vi "ask_model_core.vi"(0 "agent_simple_qa in":refnum<class "agent_simple_qa.lvclass">, 5 "message":refnum<class "abstract_message_base.lvclass">, 11 "error in (no error)":errorcluster) -> (4 "agent_simple_qa out":refnum<class "agent_simple_qa.lvclass">, 6 "message_response":refnum<class "abstract_message_base.lvclass">, 15 "error out":errorcluster)   [LabVIEW 2020, in "agent_simple_qa.lvclass"]
uses:
  agent_simple_qa.lvclass
  models/abstract_message_base/abstract_message_base.lvclass
  agent_simple_qa.lvclass/agent_simple_qa.ctl
  models/abstract_llm_chatcompletion/abstract_llm_chatcompletion.lvclass
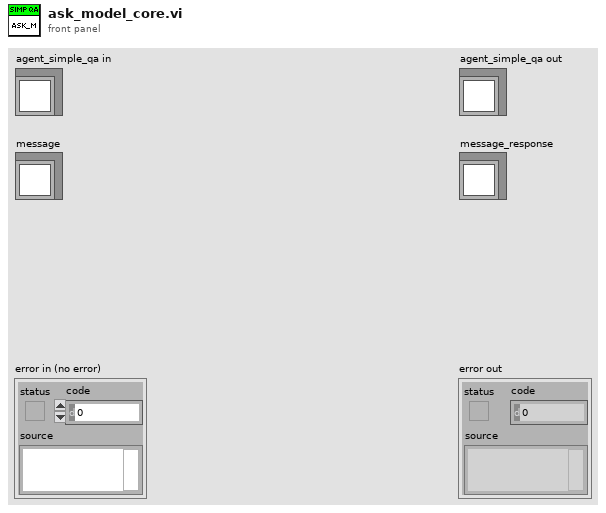
[diagram p1: front panel]
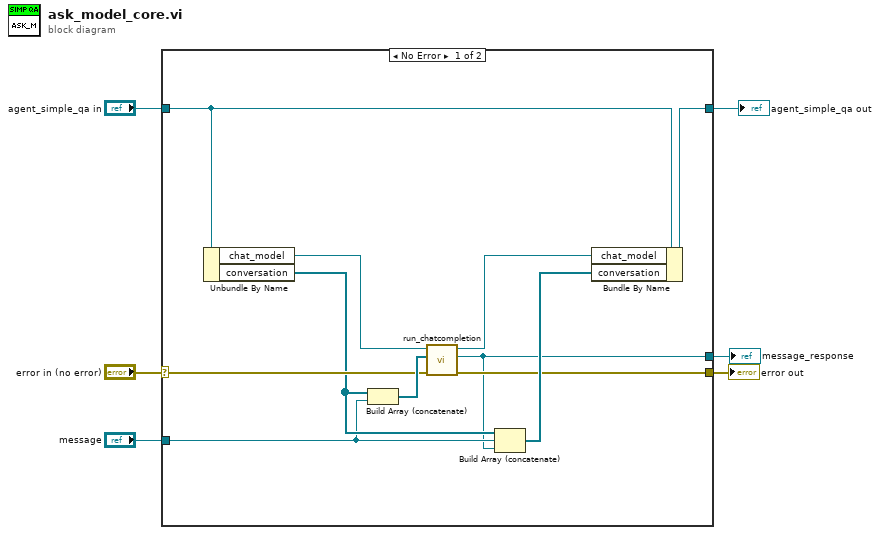
[diagram p0: block diagram]
diagram:
  n1 = case shown="No Error" "error in (no error)" {
    selector: "error in (no error)" -> [w13 w19]
    tunnel: [w8 w19] -> w5
    tunnel: [w16 w18] -> w3
    tunnel: "agent_simple_qa in" -> [w11 w18]
    tunnel: "message" -> [w9 _]
    tunnel: [w7 _] -> w2
    frame No Error {
      n2 = Unbundle By Name(w11) -> ("chat_model"=w12:refnum<class "abstract_llm_base.lvclass">, "conversation"=w10:refnum<class "abstract_message_base.lvclass">[])
      n3 = Build Array (concatenate)(w10, w9) -> (w15:refnum<class "abstract_message_base.lvclass">[])
      n4 = call "run_chatcompletion.vi"("error in (no error)"=w13, "Messages"=w15, "abstract_llm_chatcompletion in"=w12) -> ("error out"=w8:errorcluster, "Response"=w7:refnum<class "abstract_message_base.lvclass">, "abstract_llm_chatcompletion out"=w17:refnum<class "abstract_llm_base.lvclass">)  [unwired: 6 in]
      n5 = Build Array (concatenate)(w10, w9, w7) -> (w14:refnum<class "abstract_message_base.lvclass">[])
      n6 = Bundle By Name(cluster=w11, "chat_model"=w17, "conversation"=w14) -> (w16:refnum<class "agent_simple_qa.lvclass">)
    }
    frame Error {
    }
  }
  "error out" <- w5
  "agent_simple_qa out" <- w3
  "message_response" <- w2
